vi "Get Model.vi"(8 "error in (no error)":errorcluster, 11 "Simulated Scope in":refnum<class "Simulated Scope.lvclass">) -> (0 "error out":errorcluster, 2 "Model":string, 3 "Simulated Scope out":refnum<class "Simulated Scope.lvclass">)   [LabVIEW 2020, in "Simulated Scope.lvlib" / "Simulated Scope.lvclass"]
uses:
  Simulated Scope.lvclass
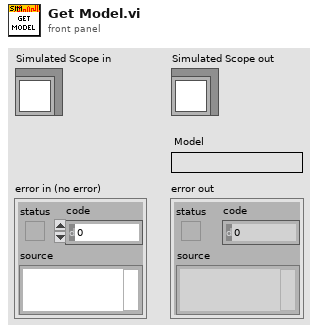
[diagram p1: front panel]
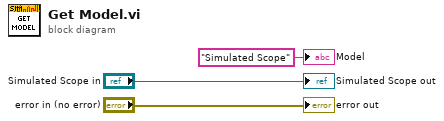
[diagram p0: block diagram]
diagram:
  "error out" <- "error in (no error)"
  "Simulated Scope out" <- "Simulated Scope in"
  "Model" <- "Simulated Scope" ("Model")
